vi "Esercizio lezione 8-1 My Simple Server.vi"(2 "stop":bool, 3 "INVIA STRINGA":bool, 4 "String in":string, 5 "Port":u16=6340) -> (0 "remote port":u16, 1 "rem addr":string)   [LabVIEW 2012]
doc: "© Copyright M. Ferrari 2010"
panel:
  # "SERVER: invia una stringa al Client"
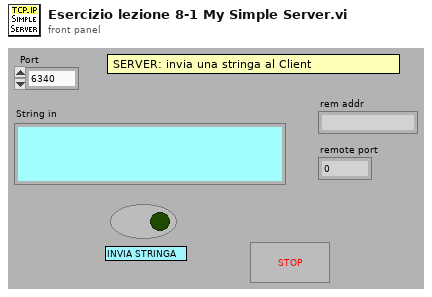
[diagram p1: front panel]
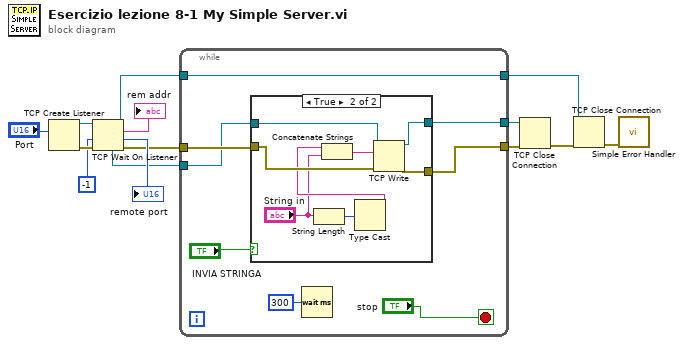
[diagram p0: block diagram]
diagram:
  n1 = TCP Create Listener(10:"Port") -> (0:w9:errorcluster, 3:w10:refnum<k5>)  [unwired: 4 in, 1 out]
  n2 = TCP Wait On Listener(8:w9, 9:-1 ("timeout ms (wait forever: -1)"), 11:w10) -> (0:w8:errorcluster, 1:→"remote port":u16, 2:→"rem addr":string, 3:w6:refnum<k5>, 4:w7:refnum<k5>)  [unwired: 1 in]
  n3 = while {
    tunnel: [w15] -> w4
    tunnel: [w18] -> w5
    tunnel: w6 -> [w18]
    tunnel: w7 -> [w19]
    tunnel: w8 -> [w20]
    tunnel: [w16] -> w13
    stop <- "stop" stop-if-true
    n4 = case shown="True" "INVIA STRINGA" {
      tunnel: w20 -> [w23 w30]
      tunnel: w19 -> [w24 w32]
      tunnel: [w24 w31] -> w16
      tunnel: [w23 w29] -> w15
      frame False {
      }
      frame True {
        n5 = String Length(string="String in") -> (length=w28:i32)
        n6 = Type Cast(x=w28) -> (*(type *) &x=w27:string)  [unwired: 1 in]
        n7 = Concatenate Strings(w27, "String in") -> (w26:string)
        n8 = TCP Write(connection ID=w32, data in=w26, error in (no error)=w30) -> (connection ID out=w31:refnum<k5>, error out=w29:errorcluster)  [unwired: 1 in, 1 out]
      }
    }
    n9 = Wait (ms)(milliseconds to wait=u32 300) -> ()  [unwired: 1 out]
  }
  n10 = TCP Close Connection(connection ID=w13, error in (no error)=w4) -> (error out=w2:errorcluster)  [unwired: 1 in, 1 out]
  n11 = TCP Close Connection(connection ID=w5, error in (no error)=w2) -> (error out=w1:errorcluster)  [unwired: 1 in, 1 out]
  n12 = call <vilib>:"Simple Error Handler.vi"("error in (no error)"=w1) -> ()  [unwired: 4 in, 5 out]
